vi "Find Project Library.vi"(8 "error in (no error)":errorcluster, 10 "library name":string, 11 "project ref":refnum<vi>) -> (0 "error out":errorcluster, 2 "found?":bool, 3 "library ref":refnum<vi>)   [LabVIEW 2017, in "Build Automation.lvlib"]
uses:
  Build Automation.lvlib
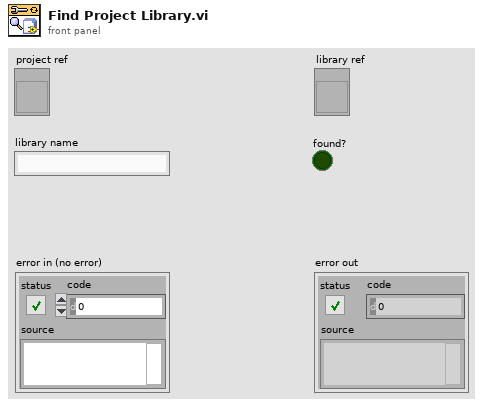
[diagram p1: front panel]
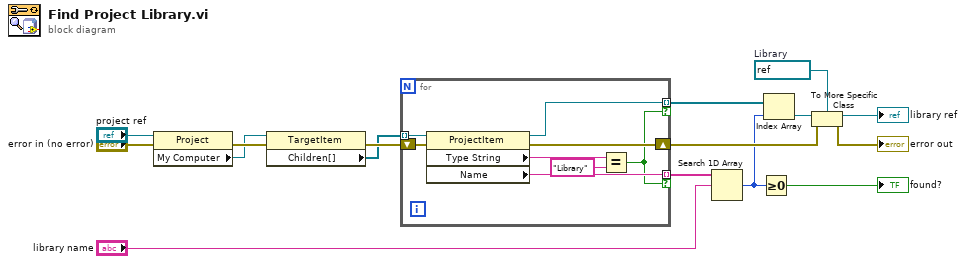
[diagram p0: block diagram]
diagram:
  w7 = refnum<vi> refnum  # Library
  n1 = property class="Project"(reference="project ref", error in="error in (no error)") -> (error out=w16:errorcluster, "My Computer"=w14:refnum<vi>)  [unwired: 1 out]
  n2 = property class="TargetItem"(reference=w14, error in=w16) -> (error out=w15:errorcluster, "Children[]"=w8:refnum<vi>[])  [unwired: 1 out]
  n3 = for {
    tunnel: w8 -> [w24] mode=indexing
    tunnel: [w18] -> w11 mode=indexing if=w17
    tunnel: [w22] -> w13 mode=indexing if=w17
    shift-right: [w20] -> w5
    shift-left: w15 -> [w21]
    n4 = property class="ProjectItem"(reference=w24, error in=w21) -> (reference out=w18:refnum<vi>, error out=w20:errorcluster, "Type String"=w19:string, "Name"=w22:string)
    n5 = Equal?(x=w19, y="Library") -> (x = y?=w17:bool)
  }
  n6 = Search 1D Array(1D array=w13, element="library name") -> (index of element=w2:i32)  [unwired: 1 in]
  n7 = Greater Or Equal To 0?(x=w2) -> (x >= 0?=→"found?":bool)
  n8 = Index Array(array=w11, index=w2) -> (element=w6:refnum<vi>)
  n9 = To More Specific Class(target class=w7, reference=w6, error in=w5) -> (specific class reference=→"library ref":refnum<vi>, error out=→"error out":errorcluster)
